vi "ex_CreateXArray.vi"(4 "time format":string, 5 "delta x":dbl format="%.2p", 6 "x0":timestamp format="%<%X\n%x>T", 7 "samples":i32) -> (2 "x array":string[](array[string]))   [LabVIEW 2017]
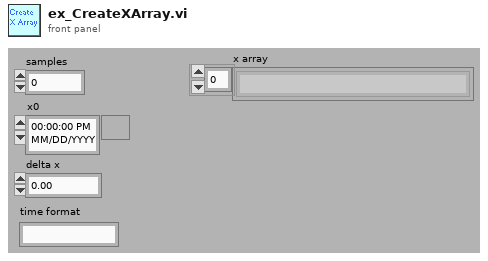
[diagram p1: front panel]
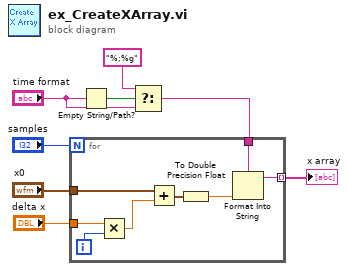
[diagram p0: block diagram]
diagram:
  n1 = Empty String/Path?(string/path="time format") -> (empty?=w4:bool)
  n2 = Select(t="%;%g" ("format string"), s=w4, f="time format") -> (s? t:f=w1:string)
  n3 = for {
    N: "samples" -> [_]
    tunnel: "x0" -> [w14]
    tunnel: "delta x" -> [w15]
    tunnel: [w12] -> w5 mode=indexing
    tunnel: w1 -> [w11]
    i -> [w16]
    n4 = Multiply(x=w15, y=w16) -> (x*y=w13:dbl)
    n5 = Add(x=w14, y=w13) -> (x+y=w9:timestamp)
    n6 = To Double Precision Float(number=w9) -> (double precision float=w10:dbl)
    n7 = Format Into String(format string=w11, w10) -> (resulting string=w12:string)  [unwired: 2 in, 1 out]
  }
  "x array" <- w5
